vi "Actor.vi"(4 "Debug Alias":string, 6 "Open Actor Core front panel? (F)":bool, 7 "error feedback":refnum<queue>, 9 "Actor":refnum<class "Actor.lvclass">, 10 "queue of queues":refnum<queue>, 11 "Message Enqueuer":refnum<class "Message Enqueuer.lvclass">) -> ()   [LabVIEW 2017, in "Actor Framework.lvlib" / "Actor.lvclass"]
doc: "(<B>Filename</B>: Actor Framework.lvlib:Actor.lvclass:Actor.vi)\n\nActor.vi is the top-level VI that is launched to be the functional aspect of the actor object. It is a wrapper around Actor Core.vi, which is where the actor defines most of its specific behavior. Actor.vi takes care of creating the caller-to-actor queue and brokering the exchange of enqueuers with the caller. It also handles all the cleanup when Actor Core.vi completes. It is not dynamic dispatch -- users of the actor framework generally don't need to understand what's being done in this function."
uses:
  Actor.lvclass
  Message Enqueuer/Message Enqueuer.lvclass
  Message Enqueuer/Message Enqueuer.lvclass/Message Enqueuer.ctl
  Actor.lvclass/Actor.ctl
  LastAck/Last Ack.lvclass/Last Ack.ctl
  Message Enqueuer/Enqueue Critical.vi
  LastAck/Last Ack.lvclass
  C:/LabVIEW Packages/Sources/PPLs/source/ActorFramework/Message/Message.lvclass
  Message Priority Queue/Priority Enqueue.vi
  Message/Message.lvclass
  Message Priority Queue/Message Priority Queue.lvclass
panel:
  out "error out":errorcluster
  # "The error out is here only as an aid to debugging if necessary."
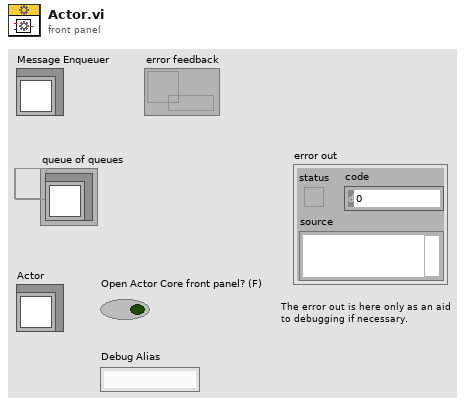
[diagram p1: front panel]
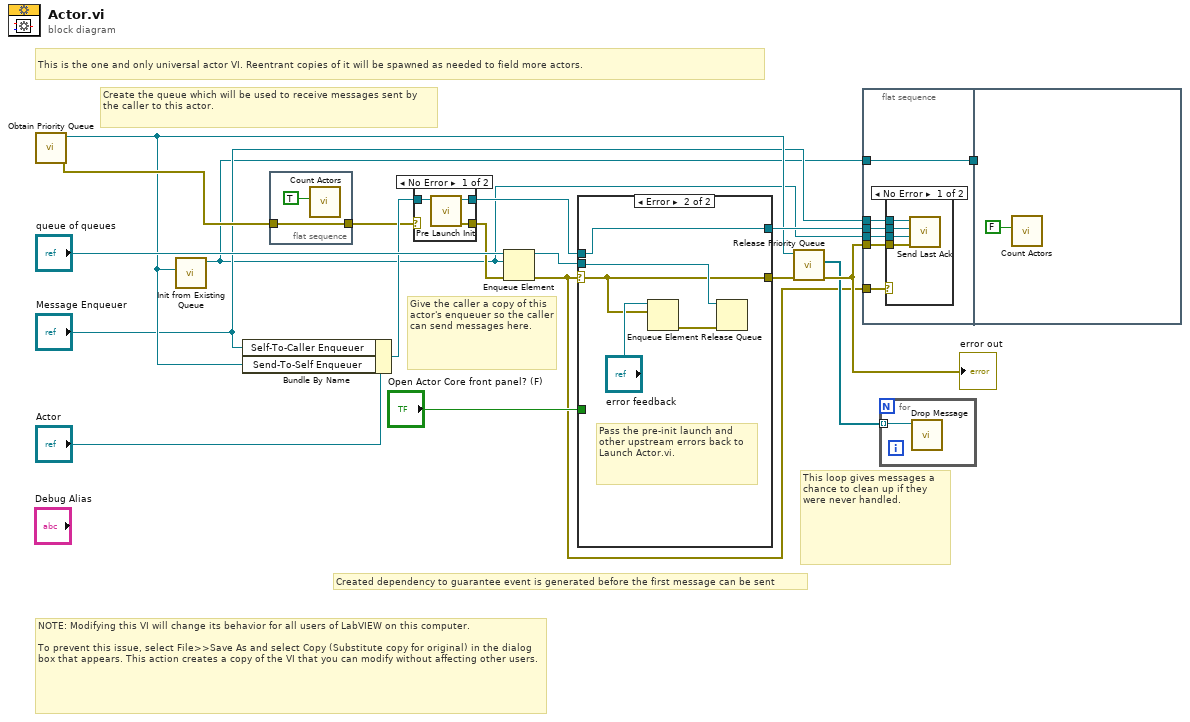
[diagram p0: block diagram]
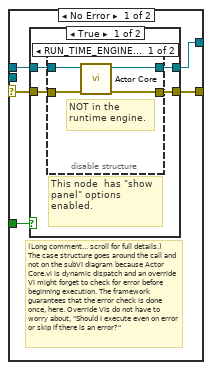
[diagram p4: hidden frame]
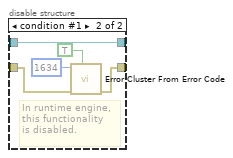
[diagram p5: hidden frame]
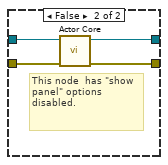
[diagram p6: hidden frame]
diagram:
  # "Created dependency to guarantee event is generated before the first message can be sent"
  # "NOTE: Modifying this VI will change its behavior for all users of LabVIEW on this computer.\n\nTo prevent this issue, select File>>Save As and select Copy (Substitute copy for original) in the dialog box that appears. This action creates a copy of the VI that you can modify without affecting other users."
  # "This loop gives messages a chance to clean up if they were never handled."
  # "Give the caller a copy of this actor's enqueuer so the caller can send messages here."
  # "Create the queue which will be used to receive messages sent by the caller to this actor."
  # "This is the one and only universal actor VI. Reentrant copies of it will be spawned as needed to field more actors."
  n1 = call "Obtain Priority Queue.vi"() -> ("error out"=w7:errorcluster, "Priority Queue"=w6:refnum<class "Message Priority Queue.lvclass">)  [unwired: 10 in]
  n2 = call "Init from Existing Queue.vi"("Priority Queue"=w6) -> ("Message Enqueuer"=w2:refnum<class "Message Enqueuer.lvclass">)  [unwired: 10 in]
  n3 = Bundle By Name(cluster="Actor", "Self-To-Caller Enqueuer"="Message Enqueuer", "Send-To-Self Enqueuer"=w6) -> (w13:refnum<class "Actor.lvclass">)
  n4 = flat-sequence {
    tunnel: [w19] -> w8
    tunnel: w7 -> [w19]
    frame #0 {
      n5 = call "Count Actors.vi"("Increment?"=TRUE) -> ()  [unwired: 11 in]
    }
  }
  n6 = case shown="No Error" w8 {
    selector: w8 -> [_ w25]
    tunnel: w13 -> [w23 w24]
    tunnel: [w22 w24] -> w12
    tunnel: [w21 w25] -> w9
    frame No Error {
      n7 = call-dynamic "Pre Launch Init.vi"("Actor in"=w23) -> ("error out"=w21:errorcluster, "Actor out"=w22:refnum<class "Actor.lvclass">)  [unwired: 9 in]
    }
    frame Error {
    }
  }
  n8 = Enqueue Element(queue="queue of queues", element=w2, error in (no error)=w9) -> (queue out=w11:refnum<queue>, error out=w1:errorcluster)  [unwired: 1 in, 1 out]
  n9 = case shown="Error" w1 {
    selector: w1 -> [w27 w48]
    tunnel: w12 -> [w28 w52]
    tunnel: [w30 w48] -> w18
    tunnel: [w29 w52] -> w16
    tunnel: w11 -> [_ w51]
    tunnel: "Open Actor Core front panel? (F)" -> [w26 _]
    frame No Error {
      # "(Long comment... scroll for full details.)\nThe case structure goes around the call and not on the subVI diagram because Actor Core.vi is dynamic dispatch and an override VI might forget to check for error before beginning execution. The framework guarantees that the error check is done once, here. Override VIs do not have to worry about, \"Should I execute even on error or skip if there is an error?\""
      n10 = case shown="True" w26 {
        tunnel: [w34 w47] -> w30
        tunnel: [w33 w46] -> w29
        tunnel: w28 -> [w32 w45]
        tunnel: w27 -> [w31 w44]
        frame True {
          # "This node  has \"show panel\" options enabled."
          n11 = disable-structure shown="RUN_TIME_ENGINE==False" {
            disable-tunnel: [w38 w42] -> w34
            disable-tunnel: [w37 w43] -> w33
            disable-tunnel: w32 -> [w36 w43]
            disable-tunnel: w31 -> [w35 w41]
            frame condition #0 (active) {
              # "NOT in the \nruntime engine."
              n12 = call-dynamic "Actor Core.vi"("error in"=w35, "Actor in"=w36) -> ("error out"=w38:errorcluster, "Actor out"=w37:refnum<class "Actor.lvclass">)  [unwired: 8 in]
            }
            frame condition #1 {
              # "In runtime engine,\nthis functionality\nis disabled."
              n13 = call <vilib>:"Error Cluster From Error Code.vi"("show call chain? (False)"=TRUE, "error in (no error)"=w41, "error code (0)"=1634) -> ("error out"=w42:errorcluster)  [unwired: 6 in]
            }
          }
        }
        frame False {
          # "This node  has \"show panel\" options disabled."
          n14 = call-dynamic "Actor Core.vi"("error in"=w44, "Actor in"=w45) -> ("error out"=w47:errorcluster, "Actor out"=w46:refnum<class "Actor.lvclass">)  [unwired: 8 in]
        }
      }
    }
    frame Error {
      # "Pass the pre-init launch and other upstream errors back to Launch Actor.vi."
      n15 = Enqueue Element(queue="error feedback", element=w48) -> (error out=w49:errorcluster)  [unwired: 2 in, 2 out]
      n16 = Release Queue(queue=w51, error in (no error)=w49) -> ()  [unwired: 1 in, 3 out]
    }
  }
  n17 = call "Release Priority Queue.vi"("error in (no error)"=w18, "Priority Queue"=w6) -> ("error out"=w17:errorcluster, "remaining elements"=w14:refnum<class "Message.lvclass">[])  [unwired: 8 in]
  "error out" <- w17
  n18 = flat-sequence {
    tunnel: w17 -> [w58]
    tunnel: w16 -> [w57]
    tunnel: "Message Enqueuer" -> [w56]
    tunnel: w2 -> [w55]
    tunnel: [w54] -> w4
    tunnel: w2 -> [w54]
    tunnel: w1 -> [w53]
    tunnel: w4 -> [_]
    frame #0 {
      n19 = case shown="No Error" w53 {
        tunnel: w58 -> [w62 _]
        tunnel: w57 -> [w61 _]
        tunnel: w56 -> [w60 _]
        tunnel: w55 -> [w59 _]
        frame No Error {
          n20 = call "Send Last Ack.vi"("error from actor"=w62, "Caller-to-Actor Enqueuer"=w59, "Actor"=w61, "Message Enqueuer"=w60) -> ()  [unwired: 8 in]
        }
        frame Error {
        }
      }
    }
    frame #1 {
      n21 = call "Count Actors.vi"("Increment?"=FALSE) -> ()  [unwired: 11 in]
    }
  }
  n22 = for {
    tunnel: w14 -> [w64] mode=indexing
    n23 = call "Drop Message.vi"("Message in"=w64) -> ()  [unwired: 11 in]
  }
